vi "E4351B_main.vi"() -> ()   [LabVIEW 2016]
doc: "Programs an SAS list for channel 1, set the transient trigger to increment it continuously, and set the data logger to take continuous measurements of channel 1's output. Finally, channel 1's voltage and curent outputs are displayed using charts."
uses:
  <vilib>/Utility/file.llb/Read Delimited Spreadsheet (DBL).vi
  <instrlib>/Agilent E4351B/Agilent E4351B.lvlib
panel:
  in  "file path":path=path "C:/Repository/bdc_prototype/logger/toVI_sec.csv"
  out "XY Graph":cluster{dbl[], dbl[]}(graph)
  out "Numeric":dbl
  out "Current":cluster{dbl[], dbl[]}(graph)
  out "Voltage":cluster{dbl[], dbl[]}(graph)
  in  "Stop VI":bool
  in  "VISA resource name":refnum<visa-resource-name>="USB0::0x0957::0x1107::MY54001612::INSTR"
  # "(c) CHANGED TOO MUCH"
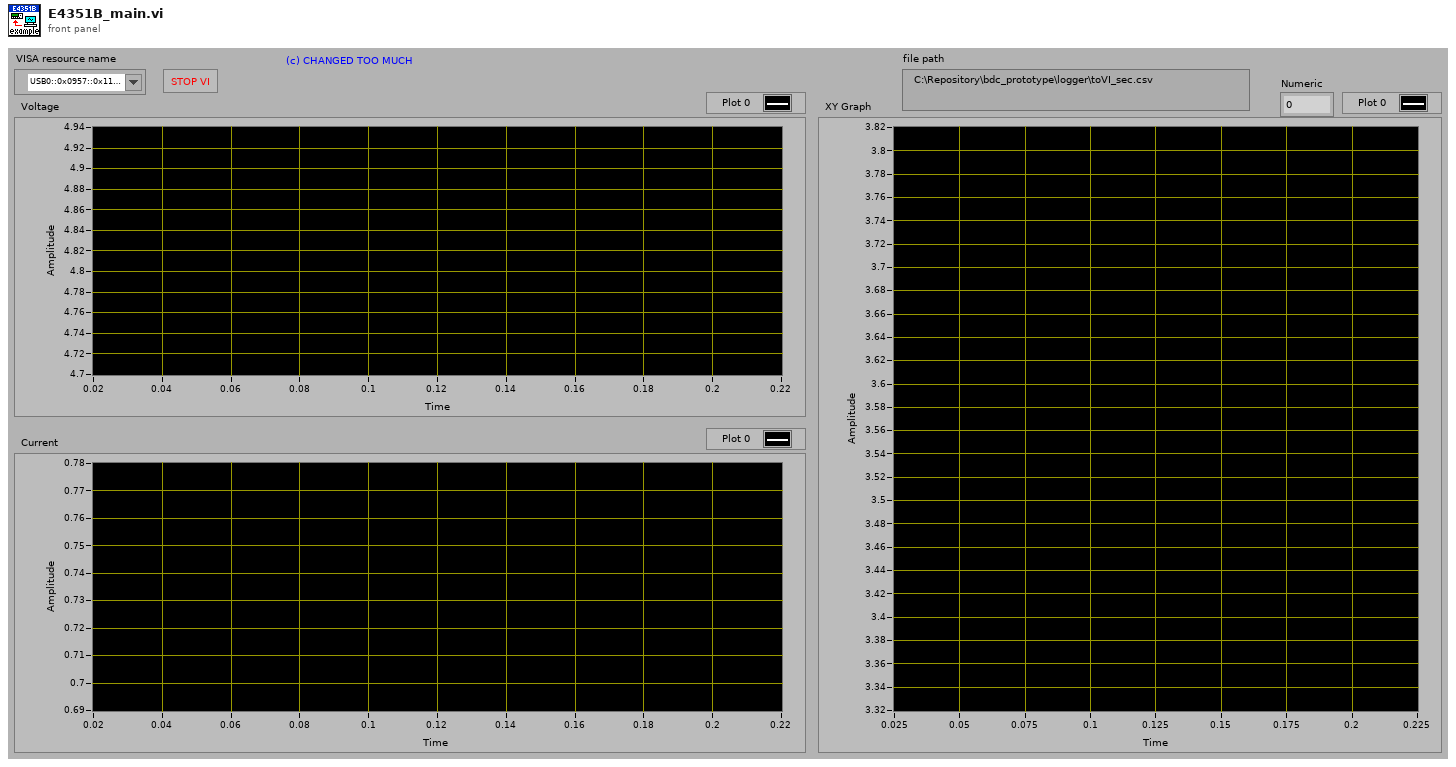
[diagram p1: front panel]
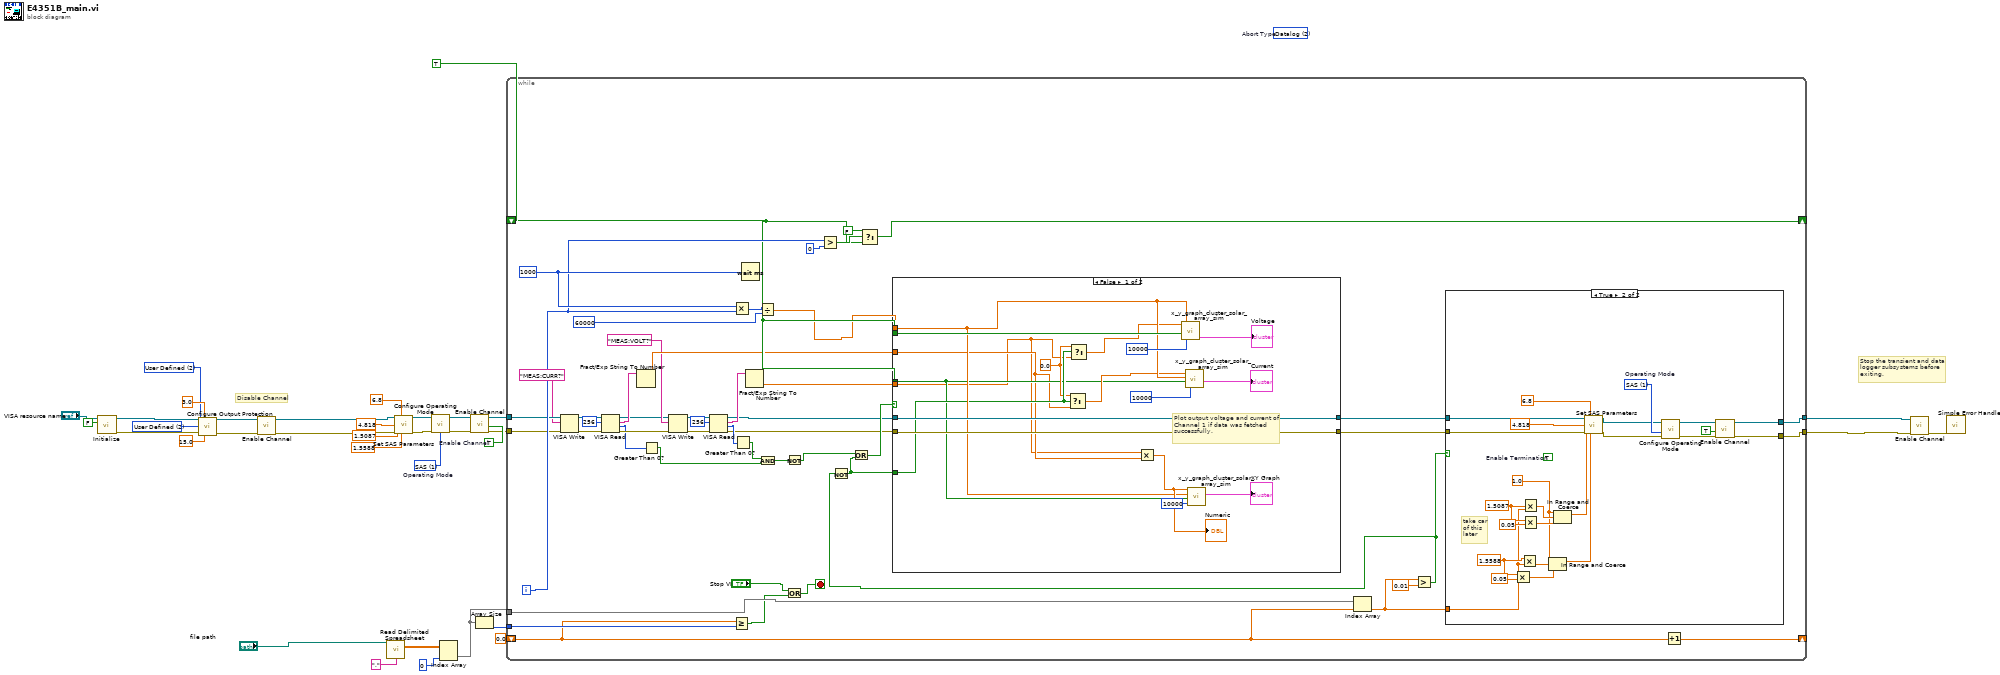
[diagram p0: block diagram]
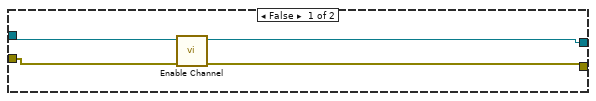
[diagram p2: hidden frame]
diagram:
  w27 = 2 items=["MAX", "MIN", "User Defined"] ("Voltage Limit Source (0:MAX)")
  w28 = 2 items=["MAX", "MIN", "User Defined"] ("Current Limit Source (0:MAX)")
  w33 = TRUE  # Enable Channel
  (unwired) 2 items=["Transient", "Acquire", "Datalog"]  # Abort Type
  w34 = 1 items=["Fixed", "SAS", "Table"]  # Operating Mode
  # "Disable Channel"
  # "Stop the transient and data logger subsystems before exiting."
  n1 = call <instrlib>:"Initialize.vi"("ID Query (True)"=FALSE, "VISA resource name"="VISA resource name") -> ("error out"=w31:errorcluster, "VISA resource name out"=w32:refnum<visa-resource-name>)  [unwired: 8 in]
  n2 = call <instrlib>:"Configure Output Protection.vi"("VISA resource name"=w32, "Current Limit (0 A)"=3.0, "Current Limit Source (0:MAX)"=w28, "Voltage Limit Source (0:MAX)"=w27, "error in (no error)"=w31, "Voltage Limit (0 V)"=15.0) -> ("VISA resource name out"=w10:refnum<visa-resource-name>, "error out"=w9:errorcluster)  [unwired: 8 in]
  n3 = call <instrlib>:"Enable Channel.vi"("error in (no error)"=w9, "VISA resource name"=w10) -> ("error out"=w25:errorcluster, "VISA resource name out"=w26:refnum<visa-resource-name>)  [unwired: 8 in]
  n4 = call-poly <vilib>:"Read Delimited Spreadsheet.vi"("file path (dialog if empty)"="file path", "delimiter (\\t)"="," ("delimiter (\\t)")) -> ("all rows"=w13:dbl[][])  [unwired: 8 in, 5 out]
  n5 = call <instrlib>:"Set SAS Parameters.vi"("VISA resource name"=w26, "Open Circuit Voltage (0.0 V)"=6.8, "Maximum Voltage Point (0.0 V)"=4.818, "Maximum Current Point (0.0 A)"=1.5087, "error in (no error)"=w25, "Short Circuit Current (0.0 A)"=1.5588) -> ("VISA resource name out"=w18:refnum<visa-resource-name>, "error out"=w17:errorcluster)  [unwired: 8 in]
  n6 = call <instrlib>:"Configure Operating Mode.vi"("error in (no error)"=w17, "Operating Mode (0:Fixed)"=w34, "VISA resource name"=w18) -> ("error out"=w7:errorcluster, "VISA resource name out"=w8:refnum<visa-resource-name>)  [unwired: 7 in]
  n7 = Index Array(array=w13, index (col)=0 ("disabled index (col)")) -> (element=w12:dbl[])  [unwired: 1 in]
  n8 = call <instrlib>:"Enable Channel.vi"("error in (no error)"=w7, "Enable Channel (Disable)"=w33, "VISA resource name"=w8) -> ("error out"=w5:errorcluster, "VISA resource name out"=w6:refnum<visa-resource-name>)  [unwired: 7 in]
  n9 = Array Size(array=w12) -> (size(s)=w11:i32)
  n10 = while {
    tunnel: w6 -> [w60]
    tunnel: [w73] -> w4
    shift-right: [w82] -> _
    shift-left: TRUE -> [w77]
    tunnel: [w72] -> w3
    shift-right: [w74] -> _
    shift-left: 0.0 -> [w36]
    tunnel: w5 -> [w59]
    tunnel: w12 -> [w71]
    tunnel: w11 -> [w68]
    i -> [w81]
    stop <- w66 stop-if-true
    w85 = u32 1000 ("milliseconds to wait")
    n11 = VISA Write(VISA resource name=w60, write buffer="MEAS:CURR?", error in (no error)=w59) -> (VISA resource name out=w56:refnum<visa-resource-name>, error out=w57:errorcluster)  [unwired: 1 out]
    n12 = VISA Read(VISA resource name=w56, byte count=u32 256, error in (no error)=w57) -> (VISA resource name out=w47:refnum<visa-resource-name>, read buffer=w54:string, return count=w43:u32, error out=w46:errorcluster)
    n13 = Fract/Exp String To Number(string=w54) -> (number=w53:dbl)  [unwired: 3 in, 1 out]
    n14 = Greater Than 0?(x=w43) -> (x > 0?=w41:bool)
    n15 = VISA Write(VISA resource name=w47, write buffer="MEAS:VOLT?", error in (no error)=w46) -> (VISA resource name out=w50:refnum<visa-resource-name>, error out=w51:errorcluster)  [unwired: 1 out]
    n16 = VISA Read(VISA resource name=w50, byte count=u32 256, error in (no error)=w51) -> (VISA resource name out=w40:refnum<visa-resource-name>, read buffer=w48:string, return count=w44:u32, error out=w39:errorcluster)
    n17 = Greater Or Equal?(x=w36, y=w68) -> (x >= y?=w65:bool)
    n18 = Multiply(x=w85, y=w81) -> (x*y=w84:u32)
    n19 = Greater Than 0?(x=w44) -> (x > 0?=w42:bool)
    n20 = Wait (ms)(milliseconds to wait=w85) -> ()  [unwired: 1 out]
    n21 = Fract/Exp String To Number(string=w48) -> (number=w45:dbl)  [unwired: 3 in, 1 out]
    n22 = Divide(x=w84, y=u32 60000) -> (x/y=w64:dbl)
    n23 = And(x=w42, y=w41) -> (x .and. y?=w38:bool)
    n24 = Not(x=w38) -> (.not. x?=w37:bool)
    n25 = Or(x="Stop VI", y=w65) -> (x .or. y?=w66:bool)
    n26 = Greater?(x=w81, y=0) -> (0:w79:bool)
    n27 = Select(t=FALSE, s=w79, f=w77) -> (s? t:f=w82:bool)
    n28 = Index Array(array=w71, index=w36) -> (element=w70:dbl)
    n29 = Greater?(x=w70, y=0.01) -> (0:w62:bool)
    n30 = Not(x=w62) -> (.not. x?=w61:bool)
    n31 = Or(x=w37, y=w61) -> (x .or. y?=w63:bool)
    n32 = case shown="False" w63 {
      tunnel: [w131 w133] -> w76
      tunnel: w40 -> [w131 w133]
      tunnel: w39 -> [w130 w132]
      tunnel: [w130 w132] -> w75
      tunnel: w64 -> [w123 _]
      tunnel: w77 -> [w125 _]
      tunnel: w77 -> [w116 _]
      tunnel: w61 -> [w118 _]
      tunnel: w53 -> [w115 _]
      tunnel: w45 -> [w114 _]
      frame False {
        w117 = 0.0 ("t")
        # "Plot output voltage and current of Channel 1 if data was fetched successfully."
        n33 = Select(t=w117, s=w118, f=w115) -> (s? t:f=w120:dbl)
        n34 = Select(t=w117, s=w118, f=w114) -> (s? t:f=w119:dbl)
        n35 = Multiply(x=w114, y=w115) -> (x*y=w124:dbl)
        "Numeric" <- w124
        n36 = call "x_y_graph_cluster_solar_array_sim.vi"("Chart History (10,000)"=10000, "Clear Graph?"=w125, "X"=w123, "Y"=w119) -> ("Cluster"=→"Voltage":cluster{dbl[], dbl[]})
        n37 = call "x_y_graph_cluster_solar_array_sim.vi"("Chart History (10,000)"=10000, "Clear Graph?"=w116, "X"=w123, "Y"=w120) -> ("Cluster"=→"Current":cluster{dbl[], dbl[]})
        n38 = call "x_y_graph_cluster_solar_array_sim.vi"("Chart History (10,000)"=10000, "Clear Graph?"=w116, "X"=w123, "Y"=w124) -> ("Cluster"=→"XY Graph":cluster{dbl[], dbl[]})
      }
      frame True {
      }
    }
    n39 = case shown="True" w62 {
      tunnel: w76 -> [w89 w112]
      tunnel: w75 -> [w87 w111]
      tunnel: [w88 w94] -> w73
      tunnel: [w86 w95] -> w72
      tunnel: w70 -> [_ w98]
      frame False {
        n40 = call <instrlib>:"Enable Channel.vi"("error in (no error)"=w87, "VISA resource name"=w89) -> ("error out"=w86:errorcluster, "VISA resource name out"=w88:refnum<visa-resource-name>)  [unwired: 8 in]
      }
      frame True {
        w90 = 1.0 ("upper limit")
        w101 = 1 items=["Fixed", "SAS", "Table"]  # Operating Mode
        w105 = 1.5588 ("Maximum Current Point (0.0 A)")
        w108 = 1.5087 ("Maximum Current Point (0.0 A)")
        (unwired) TRUE  # Enable Termination
        # "take car\nof this \nlater"
        n41 = Multiply(x=w105, y=0.05) -> (x*y=w103:dbl)
        n42 = Multiply(x=w105, y=w98) -> (x*y=w91:dbl)
        n43 = Multiply(x=w108, y=w98) -> (x*y=w92:dbl)
        n44 = Multiply(x=w108, y=0.05) -> (x*y=w106:dbl)
        n45 = In Range and Coerce(upper limit=w90, x=w91, lower limit=w103) -> (coerced(x)=w102:dbl)  [unwired: 1 out]
        n46 = In Range and Coerce(upper limit=w90, x=w92, lower limit=w106) -> (coerced(x)=w109:dbl)  [unwired: 1 out]
        n47 = call <instrlib>:"Set SAS Parameters.vi"("VISA resource name"=w112, "Open Circuit Voltage (0.0 V)"=6.8, "Maximum Voltage Point (0.0 V)"=4.818, "Maximum Current Point (0.0 A)"=w109, "error in (no error)"=w111, "Short Circuit Current (0.0 A)"=w102) -> ("VISA resource name out"=w100:refnum<visa-resource-name>, "error out"=w99:errorcluster)  [unwired: 8 in]
        n48 = call <instrlib>:"Configure Operating Mode.vi"("error in (no error)"=w99, "Operating Mode (0:Fixed)"=w101, "VISA resource name"=w100) -> ("error out"=w96:errorcluster, "VISA resource name out"=w97:refnum<visa-resource-name>)  [unwired: 7 in]
        n49 = call <instrlib>:"Enable Channel.vi"("error in (no error)"=w96, "Enable Channel (Disable)"=TRUE, "VISA resource name"=w97) -> ("error out"=w95:errorcluster, "VISA resource name out"=w94:refnum<visa-resource-name>)  [unwired: 7 in]
      }
    }
    n50 = Increment(x=w36) -> (x+1=w74:dbl)
  }
  n51 = call <instrlib>:"Enable Channel.vi"("error in (no error)"=w3, "VISA resource name"=w4) -> ("error out"=w2:errorcluster)  [unwired: 8 in, 1 out]
  n52 = call <vilib>:"Simple Error Handler.vi"("error in (no error)"=w2) -> ()  [unwired: 4 in, 5 out]
